vi "UpdateSystemNumber.vi"(0 "InSystemNo":i8=1 min=1 max=6) -> (1 "ConfigPath":path, 2 "SystemNo":i8=1 min=1 max=6, 3 "Title Block":string)   [LabVIEW 2021]
uses:
  Main Controls System v8.0/AutoAge Globals.vi
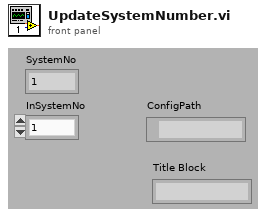
[diagram p1: front panel]
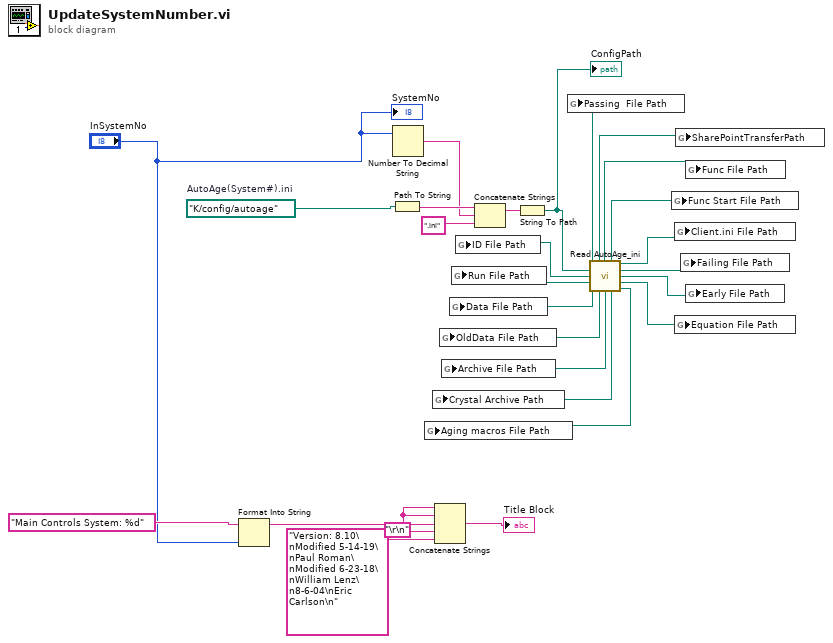
[diagram p0: block diagram]
diagram:
  w7 = "\r\n"
  w4 = path "K:/config/autoage"  # AutoAge(System#).ini
  n1 = Format Into String(format string="Main Controls System: %d", "InSystemNo") -> (resulting string=w9:string)  [unwired: 2 in, 1 out]
  n2 = Path To String(path=w4) -> (string=w27:string)
  n3 = Number To Decimal String(number="InSystemNo") -> (decimal integer string=w2:string)  [unwired: 1 in]
  n4 = Concatenate Strings(w7, w7, w9, w7, "Version: 8.10\nModified 5-14-19\nPaul Roman\nModified 6-23-18\nWilliam Lenz\n8-6-04\nEric Carlson\n") -> (→"Title Block":string)
  n5 = Concatenate Strings(w27, w2, ".ini" ("Substring")) -> (w26:string)
  n6 = String To Path(string=w26) -> (path=w5:path)
  "ConfigPath" <- w5
  n7 = call "Read AutoAge_ini.vi"("AutoAge.ini File Path"=w5) -> ("Client ini File Path"=w15:path, "Failing File Path"=w16:path, "Early File Path"=w17:path, "Equation File Path"=w18:path, "Aging Macros File Path"=w19:path, "Func Start File Path"=w14:path, "Crystal Archive File Path"=w20:path, "Func File Path"=w13:path, "Archive File Path"=w21:path, "SharePointTransferPath"=w1:path, "OldData File Path"=w22:path, "Passing File Path"=w11:path, "ID File Path"=w25:path, "Run File Path"=w24:path, "Data File Path"=w23:path)
  n8 = global write "AutoAge Globals.vi" "Aging macros File Path"(w19) -> ()
  n9 = global write "AutoAge Globals.vi" "Crystal Archive Path"(w20) -> ()
  n10 = global write "AutoAge Globals.vi" "OldData File Path"(w22) -> ()
  n11 = global write "AutoAge Globals.vi" "Archive File Path"(w21) -> ()
  n12 = global write "AutoAge Globals.vi" "Data File Path"(w23) -> ()
  n13 = global write "AutoAge Globals.vi" "Run File Path"(w24) -> ()
  n14 = global write "AutoAge Globals.vi" "ID File Path"(w25) -> ()
  n15 = global write "AutoAge Globals.vi" "Passing  File Path"(w11) -> ()
  n16 = global write "AutoAge Globals.vi" "Func Start File Path"(w14) -> ()
  n17 = global write "AutoAge Globals.vi" "Client.ini File Path"(w15) -> ()
  n18 = global write "AutoAge Globals.vi" "Equation File Path"(w18) -> ()
  n19 = global write "AutoAge Globals.vi" "SharePointTransferPath"(w1) -> ()
  n20 = global write "AutoAge Globals.vi" "Failing File Path"(w16) -> ()
  n21 = global write "AutoAge Globals.vi" "Func File Path"(w13) -> ()
  n22 = global write "AutoAge Globals.vi" "Early File Path"(w17) -> ()
  "SystemNo" <- "InSystemNo"
